vi "Get_Dusty.vi"() -> ()   [LabVIEW 2015]
uses:
  <vilib>/Utility/miscctls.llb/LVRectTypeDef.ctl
panel:
  out "error out":errorcluster
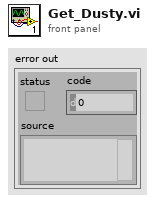
[diagram p1: front panel]
types:
  T1 = enum32{"Invalid", "Standard", "Closed", "Hidden", "Minimized", "Maximized"}
  T2 = typedef "LVRectTypeDef.ctl" = cluster{"Left":i16, "Top":i16, "Right":i16, "Bottom":i16}
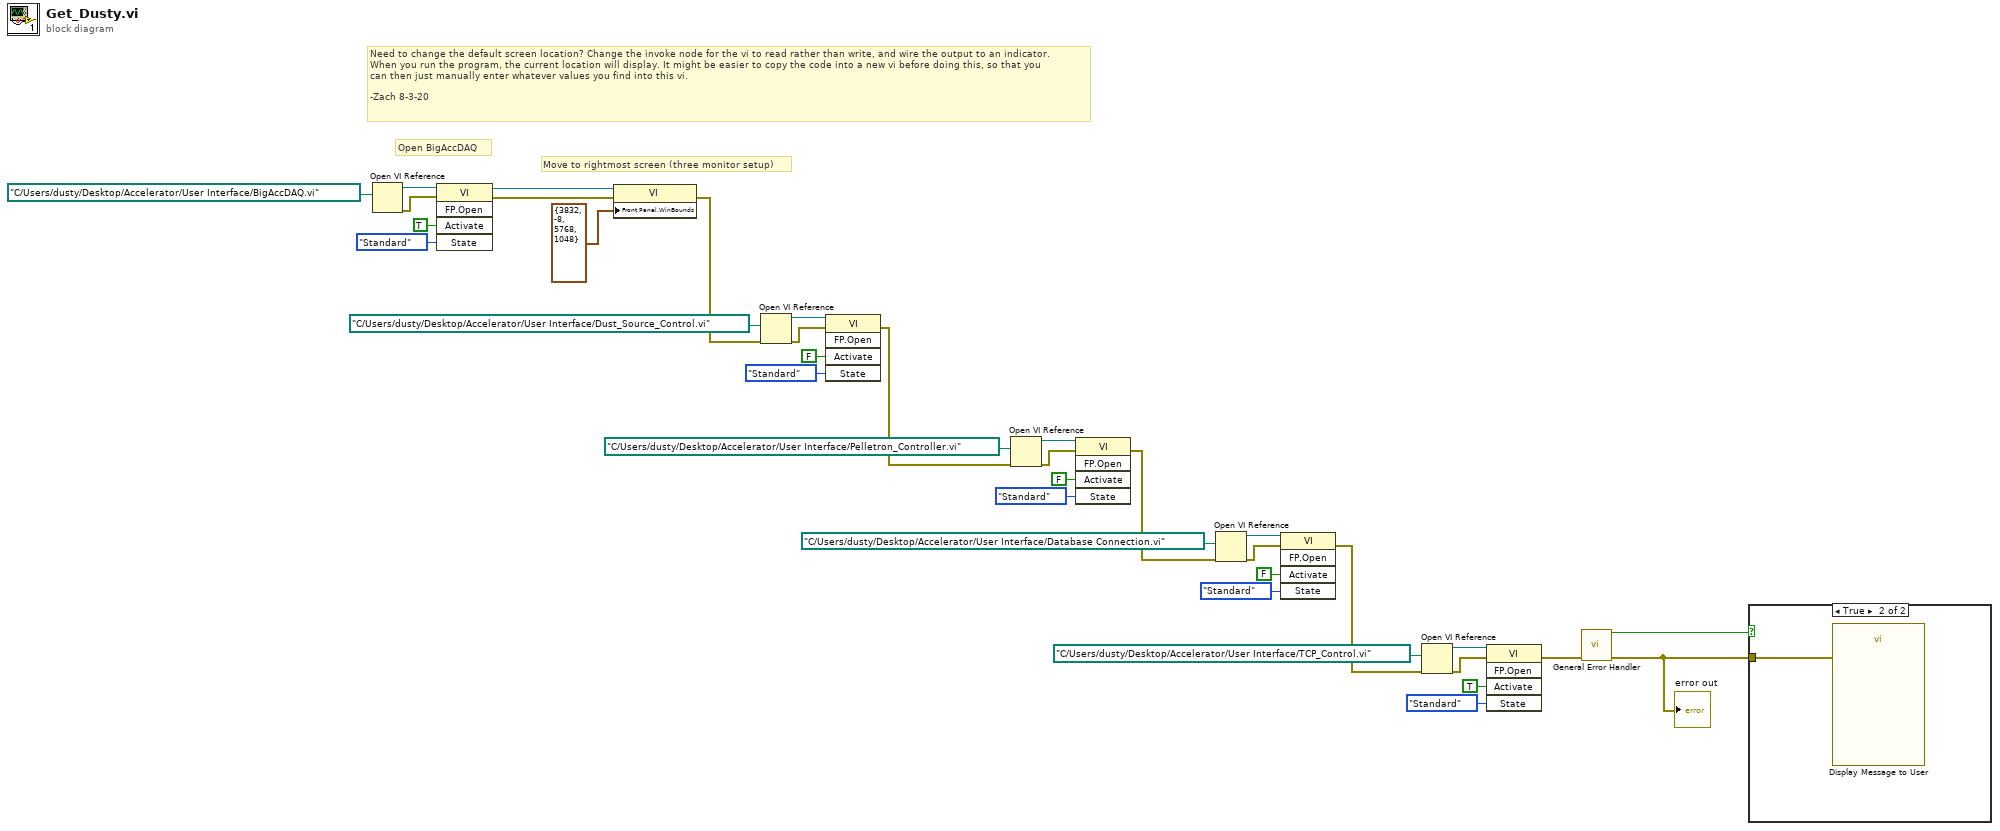
[diagram p0: block diagram]
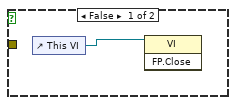
[diagram p2: hidden frame]
diagram:
  # "Need to change the default screen location? Change the invoke node for the vi to read rather than write, and wire the output to an indicator.\nWhen you run the program, the current location will display. It might be easier to copy the code into a new vi before doing this, so that you\ncan then just manually enter whatever values you find into this vi.\n\n-Zach 8-3-20"
  # "Move to rightmost screen (three monitor setup)"
  # "Open BigAccDAQ"
  n1 = Open VI Reference(vi path=path "C:/Users/dusty/Desktop/Accelerator/User Interface/BigAccDAQ.vi") -> (vi reference=w35:refnum<vi>, error out=w31:errorcluster)  [unwired: 5 in]
  n2 = invoke class="VI" method="FP.Open"(reference=w35, error in=w31, "Activate"=TRUE ("Activate?"), "State"=T1."Standard") -> (reference out=w30:refnum<vi>, error out=w29:errorcluster)  [unwired: 1 in, 3 out]
  n3 = property class="VI"(reference=w30, error in=w29, "Front Panel.WinBounds"=T2 {"Left"=3832, "Top"=-8, "Right"=5768, "Bottom"=1048} ("Front Panel Window:Window Bounds")) -> (error out=w22:errorcluster)  [unwired: 1 out]
  n4 = Open VI Reference(vi path=path "C:/Users/dusty/Desktop/Accelerator/User Interface/Dust_Source_Control.vi", error in (no error)=w22) -> (vi reference=w27:refnum<vi>, error out=w23:errorcluster)  [unwired: 4 in]
  n5 = invoke class="VI" method="FP.Open"(reference=w27, error in=w23, "Activate"=FALSE ("Activate?"), "State"=T1."Standard") -> (error out=w16:errorcluster)  [unwired: 1 in, 4 out]
  n6 = Open VI Reference(vi path=path "C:/Users/dusty/Desktop/Accelerator/User Interface/Pelletron_Controller.vi", error in (no error)=w16) -> (vi reference=w21:refnum<vi>, error out=w17:errorcluster)  [unwired: 4 in]
  n7 = invoke class="VI" method="FP.Open"(reference=w21, error in=w17, "Activate"=FALSE ("Activate?"), "State"=T1."Standard") -> (error out=w10:errorcluster)  [unwired: 1 in, 4 out]
  n8 = Open VI Reference(vi path=path "C:/Users/dusty/Desktop/Accelerator/User Interface/Database Connection.vi", error in (no error)=w10) -> (vi reference=w15:refnum<vi>, error out=w11:errorcluster)  [unwired: 4 in]
  n9 = invoke class="VI" method="FP.Open"(reference=w15, error in=w11, "Activate"=FALSE ("Activate?"), "State"=T1."Standard") -> (error out=w4:errorcluster)  [unwired: 1 in, 4 out]
  n10 = Open VI Reference(vi path=path "C:/Users/dusty/Desktop/Accelerator/User Interface/TCP_Control.vi", error in (no error)=w4) -> (vi reference=w9:refnum<vi>, error out=w5:errorcluster)  [unwired: 4 in]
  n11 = invoke class="VI" method="FP.Open"(reference=w9, error in=w5, "Activate"=TRUE ("Activate?"), "State"=T1."Standard") -> (error out=w3:errorcluster)  [unwired: 1 in, 4 out]
  n12 = call <vilib>:"General Error Handler.vi"("error in (no error)"=w3) -> ("error?"=w2:bool, "error out"=w1:errorcluster)  [unwired: 10 in, 3 out]
  "error out" <- w1
  n13 = case shown="True" w2 {
    tunnel: w1 -> [_ w37]
    frame False {
      n14 = control-ref of="This VI"() -> (w36:refnum<vi>)
      n15 = invoke class="VI" method="FP.Close"(reference=w36) -> ()  [unwired: 2 in, 3 out]
    }
    frame True {
      n16 = call "Display Message to User"("error in (no error)"=w37) -> ()  [unwired: 9 in, 2 out]
    }
  }
